vi "midichannel.get.vi"(8 "error in":errorcluster, 11 "midi in":refnum<class "midi.lvclass">) -> (0 "error out":errorcluster, 2 "midichannel":u64, 3 "midi out":refnum<class "midi.lvclass">)   [LabVIEW 2020, in "midi.lvclass"]
uses:
  midi.lvclass
  midi.lvclass/midi.ctl
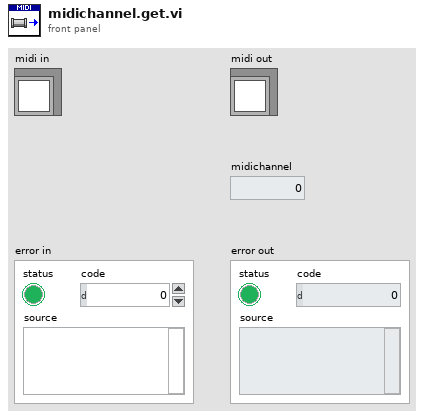
[diagram p1: front panel]
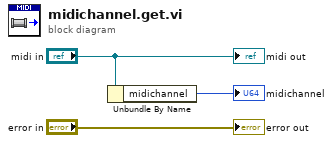
[diagram p0: block diagram]
diagram:
  n1 = Unbundle By Name("midi in") -> ("midichannel"=→"midichannel":u64)
  "midi out" <- "midi in"
  "error out" <- "error in"
